vi "Get Software Details extended.vi"(6 "Trace Component Info (F)":bool, 8 "error in (no error)":errorcluster, 11 "Software Item":u64) -> (0 "error out":errorcluster, 3 "Software Extended Info":T1 {"Visibility Type" items=["standard", "hidden", "system", "unknown", "startup", "image"]})   [LabVIEW 2012, in "nisyscfg.lvlib"]
uses:
  <vilib>/nisyscfg/nisyscfg.lvlib
  <vilib>/nisyscfg/Software Extended.ctl
  <vilib>/nisyscfg/Component Type.ctl
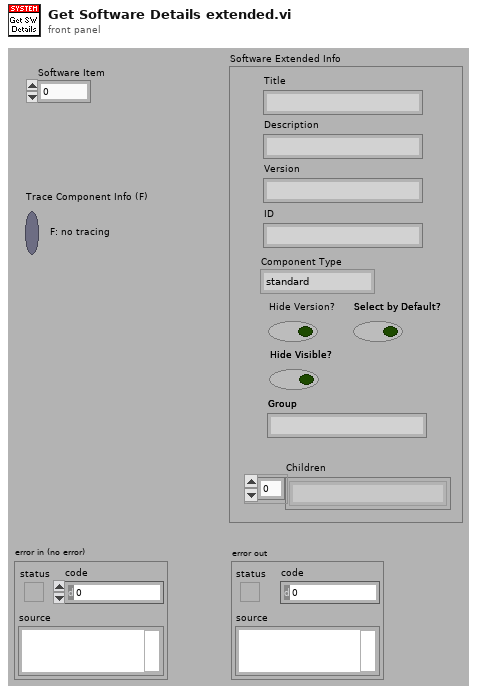
[diagram p1: front panel]
types:
  T1 = typedef "nisyscfg.lvlib/Software Extended.ctl" = cluster{"Description":string, "ID":string, "Version":string, "Title":string, "Visibility Type":T2, "Hide Version?":bool, "Children":string[], "Select by Default?":bool, "Hide Visible?":bool, "Group":string}
  T2 = typedef "nisyscfg.lvlib/Component Type.ctl" = u32
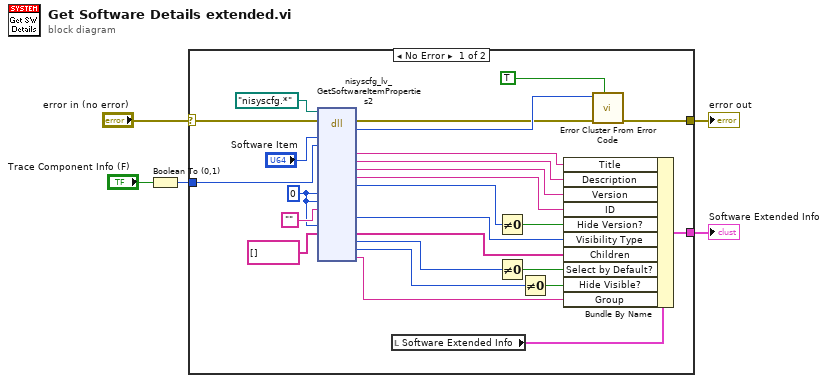
[diagram p0: block diagram]
diagram:
  n1 = Boolean To (0,1)(Boolean="Trace Component Info (F)") -> (0, 1=w1:i16)
  n2 = case shown="No Error" "error in (no error)" {
    selector: "error in (no error)" -> [w31 w32]
    tunnel: [w30 w32] -> w4
    tunnel: [w29 _] -> w3
    tunnel: w1 -> [w17 _]
    frame No Error {
      w18 = u32 0 ("isAvailable")
      n3 = dll-call lib="nisyscfg.*" fn="nisyscfg_lv_GetSoftwareItemProperties2" label="GetSoftwareItemProperties2"(path in=path "nisyscfg.*", error in=w31, "itemEnumerator"="Software Item", "logToSpy"=w17, "numChildren"=w18, "type"=w18, "oldestCompatibleVersion"="", "isAvailable"=w18, "childrenIDs"=string[] [] ("Array")) -> (error out=w27:errorcluster, "result"=w28:i32, "title"=w13:string, "description"=w12:string, "version"=w11:string, "ID"=w16:string, "hideVersion"=w25:u32, "visibilityType"=w15:u32, "childrenIDs"=w20:string[], "selectByDefault"=w10:u32, "hideVisible"=w7:u32, "group"=w6:string)  [unwired: 16 in, 1 out]
      n4 = local read "Software Extended Info"() -> (w21:T1)
      n5 = Not Equal To 0?(x=w25) -> (x != 0?=w14:bool)
      n6 = Not Equal To 0?(x=w10) -> (x != 0?=w9:bool)
      n7 = Not Equal To 0?(x=w7) -> (x != 0?=w8:bool)
      n8 = Bundle By Name(cluster=w21, "Title"=w13, "Description"=w12, "Version"=w11, "ID"=w16, "Hide Version?"=w14, "Visibility Type"=w15, "Children"=w20, "Select by Default?"=w9, "Hide Visible?"=w8, "Group"=w6) -> (w29:T1)
      n9 = call <vilib>:"Error Cluster From Error Code.vi"("show call chain? (False)"=TRUE, "error in (no error)"=w27, "error code (0)"=w28) -> ("error out"=w30:errorcluster)  [unwired: 6 in]
    }
    frame Error {
    }
  }
  "error out" <- w4
  "Software Extended Info" <- w3
